vi "sound.vi"(2 "df Array":dbl[](array[numeric]), 3 "sound?":bool, 4 "Parametros Interferometro/Freq-Volt":T1, 5 "Sound Parameters":cluster{"# samples":u32, "tiempos (ms)":dbl}, 6 "sound format":T3, 7 "Sound Device IN":cluster{"task ID":T2, "error":errorcluster} {"task ID" format="%.0x"}) -> (0 "Waveform":waveform(dbl), 1 "Sound Device OUT":cluster{"task ID":T2, "error":errorcluster} {"task ID" format="%.0x"})   [LabVIEW 2010]
uses:
  <vilib>/sound2/lvsound2.llb/Sound Data Format.ctl
  <vilib>/sound2/lvsound2.llb/Sound Output Task ID.ctl
  <vilib>/sound2/lvsound2.llb/Sound Output Write (DBL Single).vi
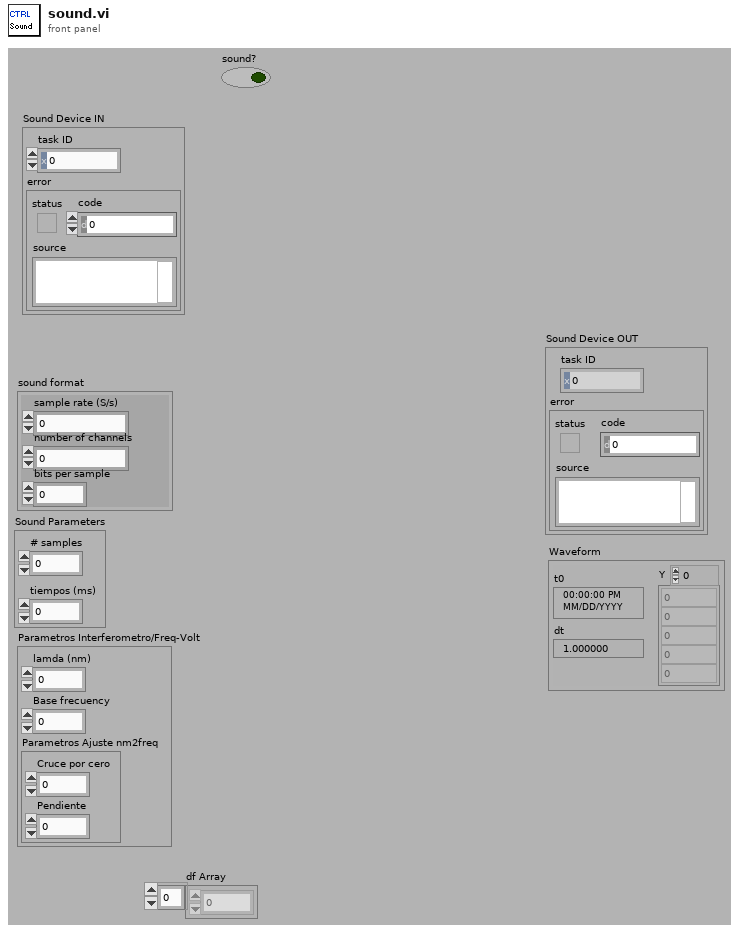
[diagram p1: front panel]
types:
  T1 = cluster{"lamda (nm)":dbl, "Base frecuency":dbl, "Parametros Ajuste nm2freq":cluster{"Cruce por cero":dbl, "Pendiente":dbl}}
  T2 = typedef "Sound Output Task ID.ctl" = u32
  T3 = typedef "Sound Data Format.ctl" = cluster{"sample rate (S/s)":dbl, "number of channels":i32, "bits per sample":i32}
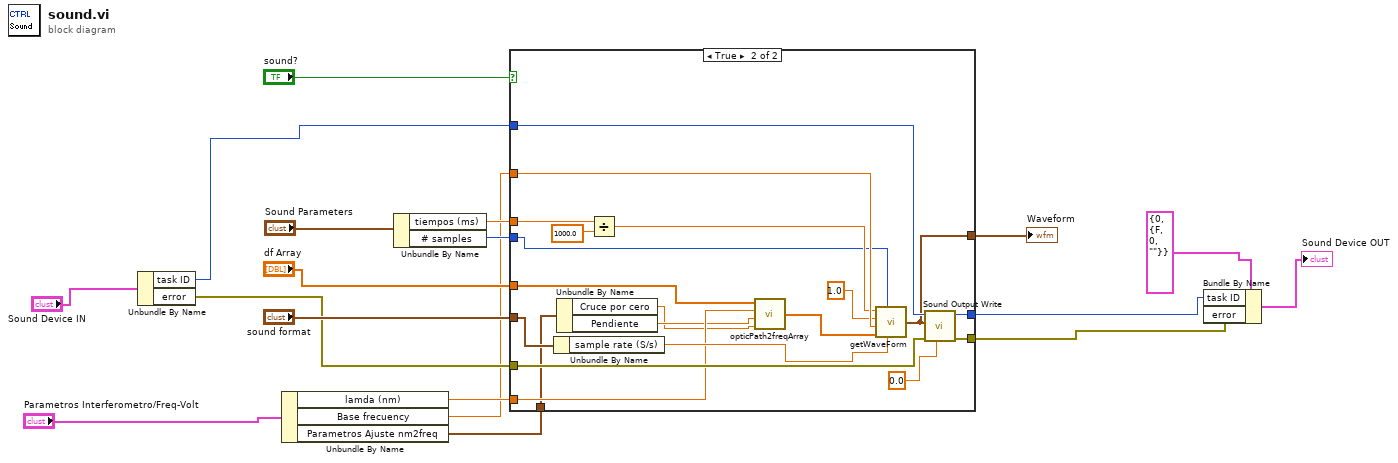
[diagram p0: block diagram]
diagram:
  n1 = Unbundle By Name("Sound Device IN") -> ("task ID"=w11:T2, "error"=w10:errorcluster)
  n2 = Unbundle By Name("Parametros Interferometro/Freq-Volt") -> ("lamda (nm)"=w3:dbl, "Base frecuency"=w2:dbl, "Parametros Ajuste nm2freq"=w1:cluster{"Cruce por cero":dbl, "Pendiente":dbl})
  n3 = Unbundle By Name("Sound Parameters") -> ("tiempos (ms)"=w14:dbl, "# samples"=w13:u32)
  n4 = case shown="True" "sound?" {
    tunnel: w11 -> [w19 w40]
    tunnel: [w19 w39] -> w6
    tunnel: w10 -> [w20 w38]
    tunnel: [w20 w37] -> w5
    tunnel: "sound format" -> [_ w35]
    tunnel: w2 -> [_ w34]
    tunnel: w14 -> [_ w31]
    tunnel: "df Array" -> [_ w22]
    tunnel: w13 -> [_ w23]
    tunnel: w3 -> [_ w28]
    tunnel: w1 -> [_ w25]
    tunnel: [_ w24] -> w15
    frame False {
    }
    frame True {
      n5 = Unbundle By Name(w35) -> ("sample rate (S/s)"=w30:dbl)
      n6 = Unbundle By Name(w25) -> ("Cruce por cero"=w26:dbl, "Pendiente"=w27:dbl)
      n7 = Divide(x=w31, y=1000.0) -> (x/y=w29:dbl)
      n8 = call "opticPath2freqArray.vi"("b"=w26, "m"=w27, "lamda (nm)"=w28, "camino optico (nm)"=w22) -> ("freq"=w21:dbl[])
      n9 = call "getWaveForm.vi"("tiempo (s)"=w29, "#samples"=w23, "Amplitud"=1.0, "frecuencia"=w34, "Fs (S/s)"=w30, "df"=w21) -> ("Waveform"=w24:waveform(dbl))  [unwired: 2 out]
      n10 = call-poly <vilib>:"Sound Output Write.vi"("timeout (sec)"=0.0, "error in (no error)"=w38, "data"=w24, "task ID"=w40) -> ("error out"=w37:errorcluster, "task ID out"=w39:T2)  [unwired: 6 in]
    }
  }
  "Waveform" <- w15
  n11 = Bundle By Name(cluster=cluster{"task ID":T2, "error":errorcluster} {"task ID"=0, "error"={"status"=FALSE, "code"=0, "source"=""}} ("Sound Device 2"), "task ID"=w6, "error"=w5) -> (→"Sound Device OUT":cluster{"task ID":T2, "error":errorcluster})
